vi "CSMKVMap-Preview.vi"(6 "Error in":errorcluster caption="Error in (no error)") -> (0 "Error out":errorcluster, 3 "Array":cluster{string, variant}[](array[cluster]))   [LabVIEW 2017, in "Communicable State Machine.lvlib"]
uses:
  Communicable State Machine.lvlib
  CSMKVMapDVR.vi
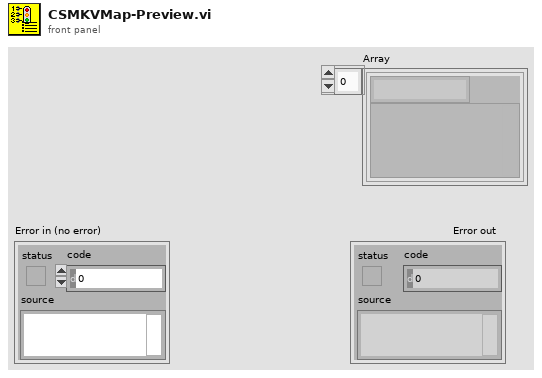
[diagram p1: front panel]
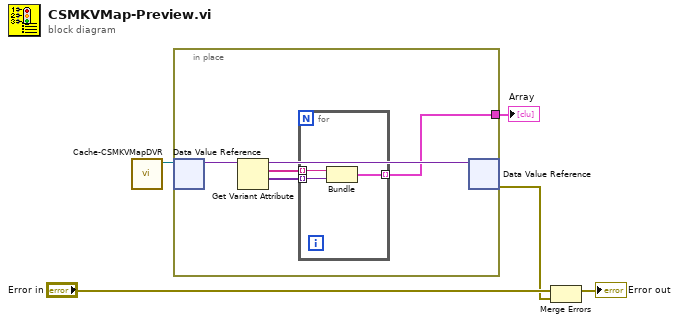
[diagram p0: block diagram]
diagram:
  n1 = call "Cache-CSMKVMapDVR.vi"() -> ("KVMapDVR"=w2:refnum<data-value>)  [unwired: 11 in]
  n2 = in-place {
    in-place-border: [w6] -> w1
    n3 = in-place-dvr #1(w2) -> (w10:variant)  [unwired: 1 out]
    n4 = Get Variant Attribute(Variant=w10) -> (duplicate Variant=w9:variant, names=w8:string[], values=w7:variant[])  [unwired: 3 in, 1 out]
    n5 = for {
      tunnel: w8 -> [w13] mode=indexing
      tunnel: w7 -> [w12] mode=indexing
      tunnel: [w11] -> w6 mode=indexing
      n6 = Bundle(w13, w12) -> (w11:cluster{string, variant})  [unwired: 1 in]
    }
    n7 = in-place-dvr #1(w9) -> (w3:errorcluster)  [unwired: 1 out]
  }
  "Array" <- w1
  n8 = Merge Errors("Error in", w3) -> (→"Error out":errorcluster)
